vi "Get Sensor Values.vi"(0 "Ref_Drive 1R":T4, 1 "Upper_Pressure_Transducer":T1={"DevStatus"={"status"=FALSE, "code"=0, "source"=""}, "Analog Channel"=enum."Invalid"}, 5 "Ref_Drive 2R":T4, 7 "Ref_Drive 4L":T4, 9 "Ref_Drive 5L":T4, 11 "Ref_Drive 6L":T4, 12 "Ref_Drive 3R":T4, 13 "Ref_Compressor":T3) -> ()   [LabVIEW 2018]
uses:
  <vilib>/Rock Robotics/WPI/MotorControl/WPI_MotorControlDeviceRef.ctl
  <vilib>/Rock Robotics/WPI/MotorControl/WPI_MotorControlType.ctl
  <vilib>/Rock Robotics/SystemInterfaces/DIO/FPGA_DIOPWMChannel.ctl
  <vilib>/Rock Robotics/WPI/PWM/WPI_PWMDeadband.ctl
  <vilib>/Rock Robotics/SystemInterfaces/DIO/FPGA_DIOChannel.ctl
  <vilib>/Rock Robotics/WPI/Compressor/WPI_CompressorDevRef.ctl
  <vilib>/Rock Robotics/WPI/AnalogChannel/WPI_AnalogChannelDevRef.ctl
  <vilib>/Rock Robotics/SystemInterfaces/AI/FPGA_AIChannel.ctl
  Sensor Readings.vi
  Robot States.vi
  CurrentMonitoring.vi
panel:
  in  "Suction_Threshold_(V)":dbl=0.1
  out "Drive Encoder Velocities":cluster{dbl, dbl}
  in  "Plot Drive Encoder Data":bool
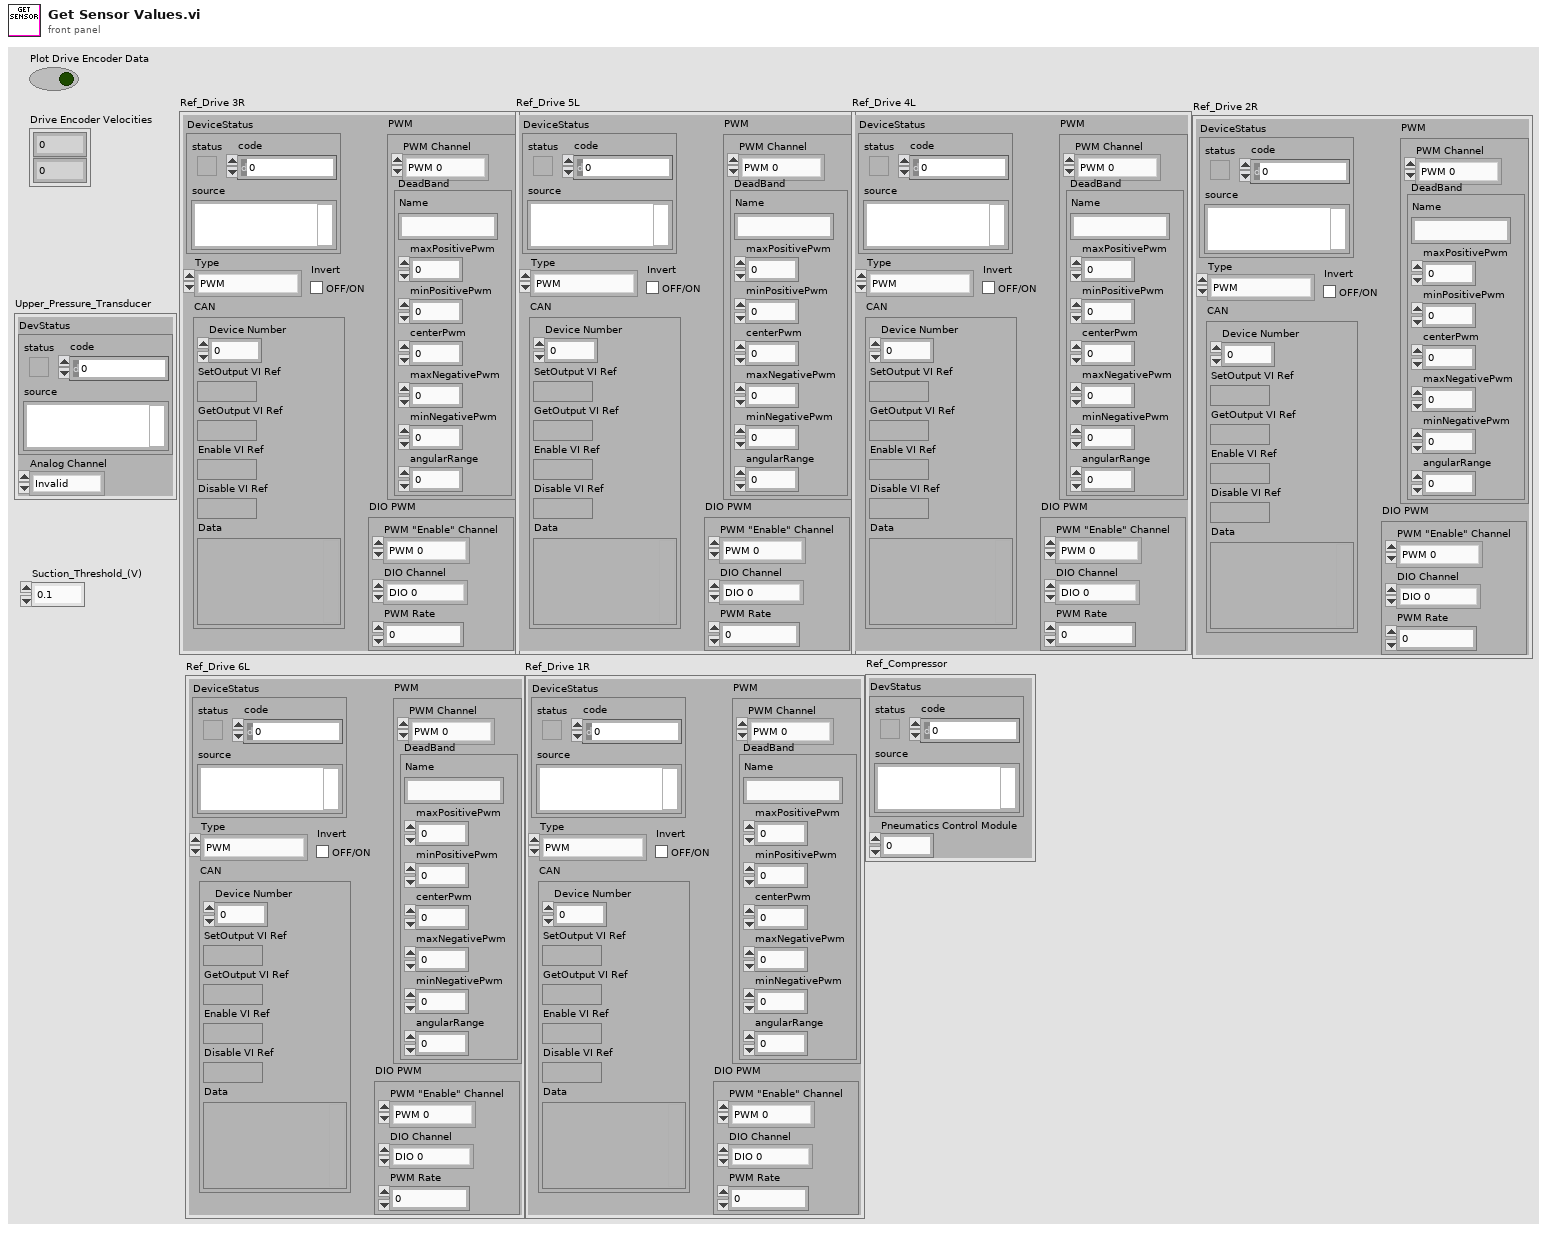
[diagram p1: front panel]
types:
  T1 = typedef "WPI_AnalogChannelDevRef.ctl" = cluster{"DevStatus":errorcluster, "Analog Channel":T2}
  T2 = typedef "FPGA_AIChannel.ctl" = enum8{"AI 0", "AI 1", "AI 2", "AI 3", "AI MXP 0", "AI MXP 1", "AI MXP 2", "AI MXP 3", "Invalid"}
  T3 = typedef "WPI_CompressorDevRef.ctl" = cluster{"DevStatus":errorcluster, "Pneumatics Control Module":u8}
  T4 = typedef "WPI_MotorControlDeviceRef.ctl" = cluster{"DeviceStatus":errorcluster, "Type":T5, "PWM":cluster{"PWM Channel":T6, "DeadBand":T7}, "CAN":cluster{"Device Number":u8, "SetOutput VI Ref":variant, "GetOutput VI Ref":variant, "Enable VI Ref":variant, "Disable VI Ref":variant, "Data":variant}, "Invert":bool, "DIO PWM":cluster{"PWM \"Enable\" Channel":T6, "DIOChannel":T8, "PWM Rate":dbl}}
  T5 = typedef "WPI_MotorControlType.ctl" = enum16{"PWM", "CAN", "DIO PWM"}
  T6 = typedef "FPGA_DIOPWMChannel.ctl" = enum8{"PWM 0", "PWM 1", "PWM 2", "PWM 3", "PWM 4", "PWM 5", "PWM 6", "PWM 7", "PWM 8", "PWM 9", "PWM MXP 0", "PWM MXP 1", "PWM MXP 2", "PWM MXP 3", "PWM MXP 4", "PWM MXP 5", "PWM MXP 6", "PWM MXP 7", "PWM MXP 8", "PWM MXP 9", "Invalid"}
  T7 = typedef "WPI_PWMDeadband.ctl" = cluster{"Name":string, "maxPositivePwm":i32, "minPositivePwm":i32, "centerPwm":i32, "maxNegativePwm":i32, "minNegativePwm":i32, "angularRange":u16}
  T8 = typedef "FPGA_DIOChannel.ctl" = enum8{"DIO 0", "DIO 1", "DIO 2", "DIO 3", "DIO 4", "DIO 5", "DIO 6", "DIO 7", "DIO 8", "DIO 9", "DIO MXP 0", "DIO MXP 1", "DIO MXP 2", "DIO MXP 3", "DIO MXP 4", "DIO MXP 5", "DIO MXP 6", "DIO MXP 7", "DIO MXP 8", "DIO MXP 9", "DIO MXP 10", "DIO MXP 11", "DIO MXP 12", "DIO MXP 13", "DIO MXP 14", "DIO MXP 15", "SPI Port CS1", "SPI Port CS2", "SPI Port CS3", "SPI Port MISO", "SPI Port MOSI", "Invalid"}
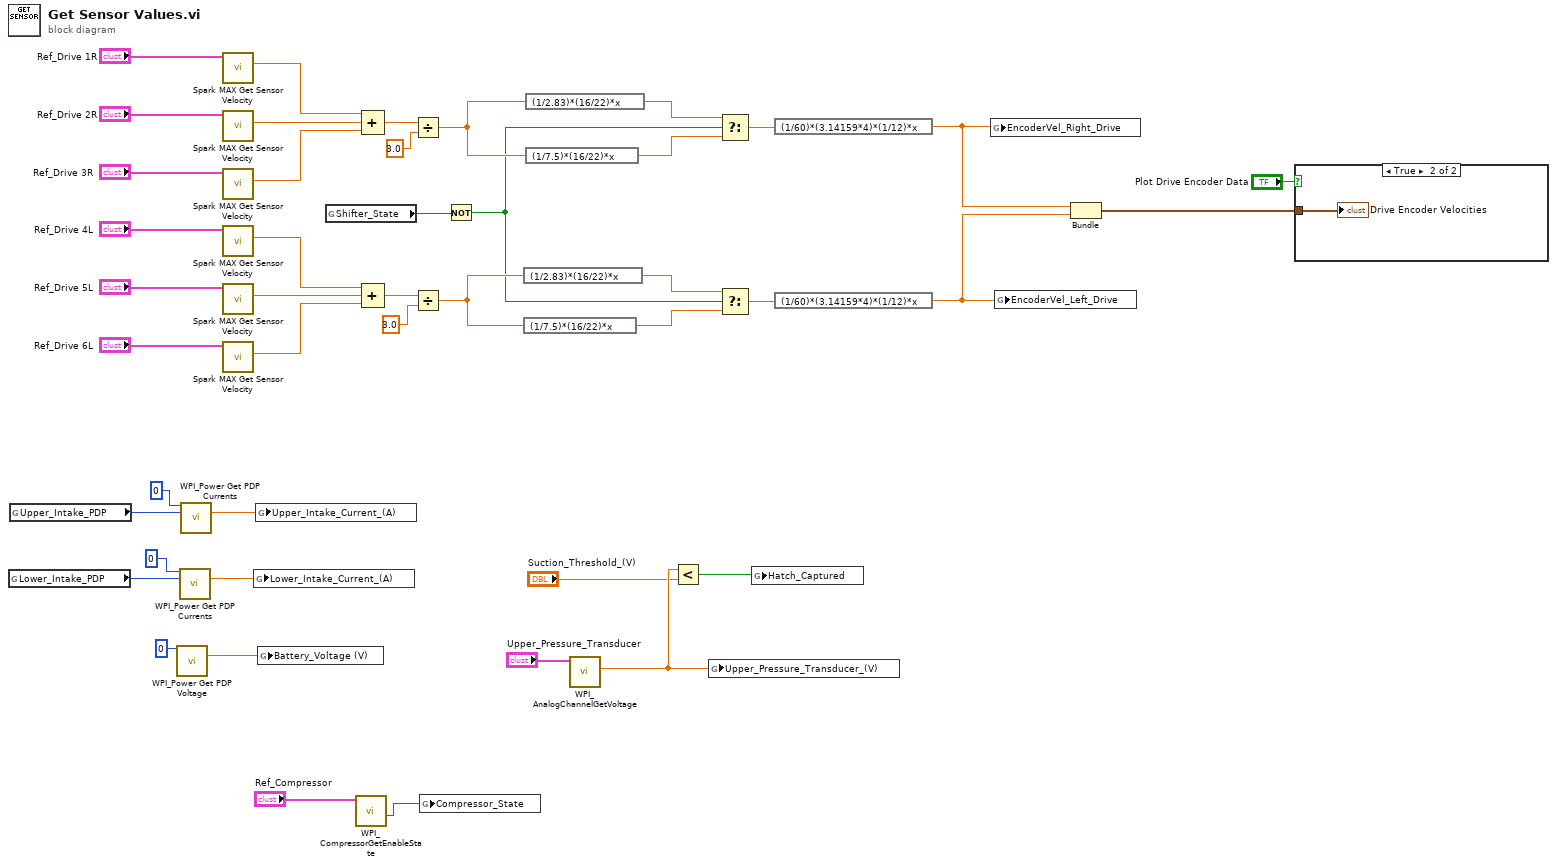
[diagram p0: block diagram]
diagram:
  n1 = global read "CurrentMonitoring.vi" "Lower_Intake_PDP"() -> (w42:i8)
  n2 = global read "CurrentMonitoring.vi" "Upper_Intake_PDP"() -> (w43:i8)
  n3 = call <vilib>:"WPI_Power Get PDP Voltage.vi"("Power Distribution Panel (0)"=u8 0) -> ("voltage (V)"=w38:dbl)  [unwired: 13 in, 1 out]
  n4 = call <vilib>:"WPI_Power Get PDP Currents.vi"("Power Distribution Panel (0)"=u8 0, "PDP Channel"=w42) -> ("current (A)"=w44:dbl)  [unwired: 11 in, 2 out]
  n5 = call <vilib>:"WPI_Power Get PDP Currents.vi"("Power Distribution Panel (0)"=u8 0, "PDP Channel"=w43) -> ("current (A)"=w39:dbl)  [unwired: 11 in, 2 out]
  n6 = call <vilib>:"Spark MAX Get Sensor Velocity.vi"("MotorControlDevRef in"="Ref_Drive 1R") -> ("Sensor Velocity"=w30:dbl)  [unwired: 7 in, 3 out]
  n7 = call <vilib>:"Spark MAX Get Sensor Velocity.vi"("MotorControlDevRef in"="Ref_Drive 2R") -> ("Sensor Velocity"=w29:dbl)  [unwired: 7 in, 3 out]
  n8 = call <vilib>:"Spark MAX Get Sensor Velocity.vi"("MotorControlDevRef in"="Ref_Drive 3R") -> ("Sensor Velocity"=w28:dbl)  [unwired: 7 in, 3 out]
  n9 = call <vilib>:"Spark MAX Get Sensor Velocity.vi"("MotorControlDevRef in"="Ref_Drive 4L") -> ("Sensor Velocity"=w27:dbl)  [unwired: 7 in, 3 out]
  n10 = call <vilib>:"Spark MAX Get Sensor Velocity.vi"("MotorControlDevRef in"="Ref_Drive 5L") -> ("Sensor Velocity"=w26:dbl)  [unwired: 7 in, 3 out]
  n11 = call <vilib>:"Spark MAX Get Sensor Velocity.vi"("MotorControlDevRef in"="Ref_Drive 6L") -> ("Sensor Velocity"=w25:dbl)  [unwired: 7 in, 3 out]
  n12 = global write "Sensor Readings.vi" "Lower_Intake_Current_(A)"(w44) -> ()
  n13 = global write "Sensor Readings.vi" "Upper_Intake_Current_(A)"(w39) -> ()
  n14 = global write "Sensor Readings.vi" "Battery_Voltage (V)"(w38) -> ()
  n15 = global read "Robot States.vi" "Shifter_State"() -> (w20:bool)
  n16 = call <vilib>:"WPI_CompressorGetEnableState.vi"("CompressorDevRef"="Ref_Compressor") -> ("Compressor Running"=w5:bool)  [unwired: 7 in, 3 out]
  n17 = Compound Arithmetic op=ADD(w30, w29, w28) -> (w22:dbl)
  n18 = Compound Arithmetic op=ADD(w27, w26, w25) -> (w21:dbl)
  n19 = Divide(x=w22, y=3.0) -> (x/y=w18:dbl)
  n20 = Divide(x=w21, y=3.0) -> (x/y=w19:dbl)
  n21 = global write "Robot States.vi" "Compressor_State"(w5) -> ()
  n22 = Not(x=w20) -> (.not. x?=w13:bool)
  n23 = expression code="(1/2.83)*(16/22)*x"(w19) -> (w15:dbl)
  n24 = expression code="(1/7.5)*(16/22)*x"(w19) -> (w14:dbl)
  n25 = expression code="(1/2.83)*(16/22)*x"(w18) -> (w17:dbl)
  n26 = expression code="(1/7.5)*(16/22)*x"(w18) -> (w16:dbl)
  n27 = call <vilib>:"WPI_AnalogChannelGetVoltage.vi"("AIDeviceRef"="Upper_Pressure_Transducer") -> ("Voltage"=w3:dbl)  [unwired: 8 in, 2 out]
  n28 = Less?(x=w3, y="Suction_Threshold_(V)") -> (x < y?=w1:bool)
  n29 = global write "Sensor Readings.vi" "Upper_Pressure_Transducer_(V)"(w3) -> ()
  n30 = Select(t=w17, s=w13, f=w16) -> (s? t:f=w12:dbl)
  n31 = Select(t=w15, s=w13, f=w14) -> (s? t:f=w11:dbl)
  n32 = global write "Sensor Readings.vi" "Hatch_Captured"(w1) -> ()
  n33 = expression code="(1/60)*(3.14159*4)*(1/12)*x"(w12) -> (w10:dbl)
  n34 = expression code="(1/60)*(3.14159*4)*(1/12)*x"(w11) -> (w9:dbl)
  n35 = global write "Sensor Readings.vi" "EncoderVel_Right_Drive"(w10) -> ()
  n36 = global write "Sensor Readings.vi" "EncoderVel_Left_Drive"(w9) -> ()
  n37 = Bundle(w10, w9) -> (w7:cluster{dbl, dbl})  [unwired: 1 in]
  n38 = case shown="True" "Plot Drive Encoder Data" {
    tunnel: w7 -> [_ w45]
    frame False {
    }
    frame True {
      "Drive Encoder Velocities" <- w45
    }
  }
